vi "Play sound.vi"() -> ()   [LabVIEW 2017]
panel:
  in  "path":path=path "D:/LabVIEW VI/LVTetris/Tetris Sounds"
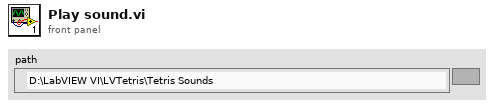
[diagram p1: front panel]
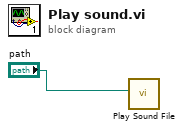
[diagram p0: block diagram]
diagram:
  n1 = call <vilib>:"Play Sound File.vi"("path"="path") -> ()  [unwired: 9 in, 2 out]
